vi "GetBoolean.vi"(6 "false string (0)":string="0", 7 "key description":string, 8 "sections":string[](array[string]), 9 "boolean":bool, 11 "info data":string) -> (0 "sections out":string[](array[string]), 1 "found?":bool, 2 "value":bool, 3 "info data out":string)   [LabVIEW 2013, in "infolib.lvlib"]
doc: "Add a new numeric key to Info Data string. If section exists in Info Data string, inserts key into this section."
uses:
  infolib.lvlib
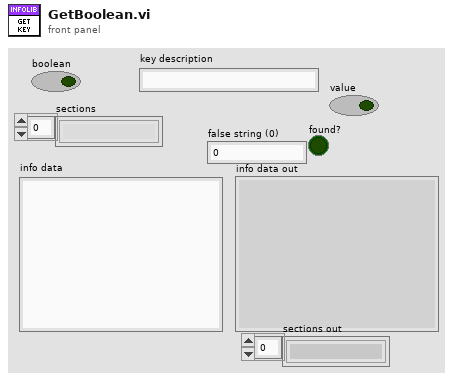
[diagram p1: front panel]
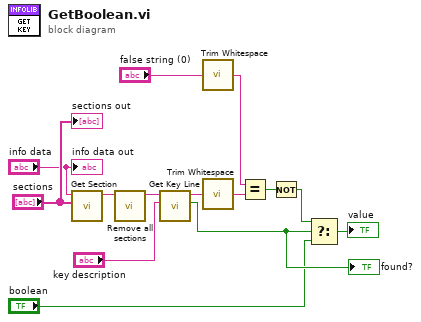
[diagram p0: block diagram]
diagram:
  n1 = call "Get Section.vi"("sections"="sections", "info data"="info data") -> ("section part"=w14:string)  [unwired: 8 in, 1 out]
  n2 = call "Remove all sections.vi"("info data"=w14) -> ("info data out"=w12:string)  [unwired: 10 in]
  n3 = call "Get Key Line.vi"("key description"="key description", "info data"=w12) -> ("found?"=w4:bool, "key value"=w6:string)  [unwired: 8 in]
  "found?" <- w4
  n4 = call <vilib>:"Trim Whitespace.vi"("string"="false string (0)") -> ("trimmed string"=w8:string)  [unwired: 1 in]
  n5 = call <vilib>:"Trim Whitespace.vi"("string"=w6) -> ("trimmed string"=w7:string)  [unwired: 1 in]
  n6 = Equal?(x=w8, y=w7) -> (x = y?=w5:bool)
  n7 = Not(x=w5) -> (.not. x?=w2:bool)
  n8 = Select(t=w2, s=w4, f="boolean") -> (s? t:f=→"value":bool)
  "info data out" <- "info data"
  "sections out" <- "sections"
